vi "Set Notifier Ref.vi"(8 "error in (no error)":errorcluster, 10 "notifier in":refnum<notifier>, 11 "CVT_DBL in":refnum<class "CVT_DBL.lvclass">) -> (0 "error out":errorcluster, 3 "CVT_DBL out":refnum<class "CVT_DBL.lvclass">)   [LabVIEW 2024, in "Current Value Table.lvlib" / "CVT_DBL.lvclass"]
uses:
  CVT_DBL.lvclass
  CVT_DBL.lvclass/CVT_DBL.ctl
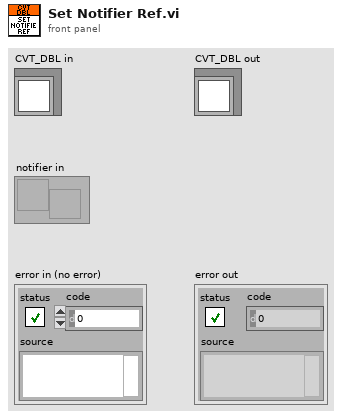
[diagram p1: front panel]
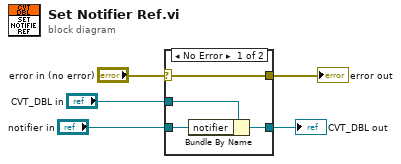
[diagram p0: block diagram]
diagram:
  n1 = case shown="No Error" "error in (no error)" {
    selector: "error in (no error)" -> [w9 w11]
    tunnel: [w9 w11] -> w4
    tunnel: [w7 w10] -> w2
    tunnel: "CVT_DBL in" -> [w8 w10]
    tunnel: "notifier in" -> [w6 _]
    frame No Error {
      n2 = Bundle By Name(cluster=w8, "notifier"=w6) -> (w7:refnum<class "CVT_DBL.lvclass">)
    }
    frame Error {
    }
  }
  "error out" <- w4
  "CVT_DBL out" <- w2
